vi "subVI_weighted_avg.vi"(9 "input array":dbl[](array[numeric]), 10 "sample":dbl, 11 "no. moving avg.":i32=5) -> (2 "weighted avg.":dbl, 3 "output array":dbl[](array[numeric]))   [LabVIEW 2018]
panel:
  out "array (last n elements first)":dbl[](array[numeric])
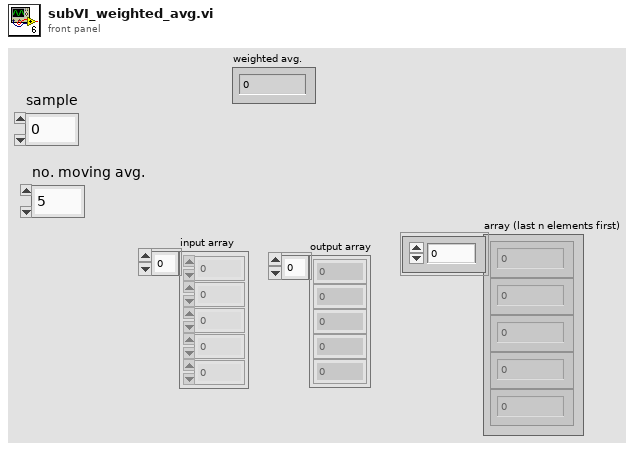
[diagram p1: front panel]
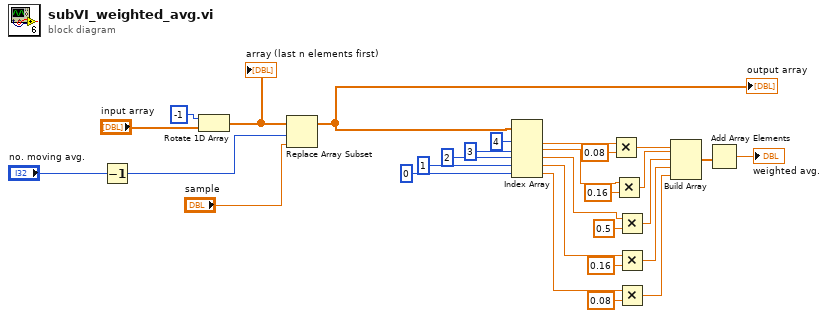
[diagram p0: block diagram]
diagram:
  n1 = Decrement(x="no. moving avg.") -> (x-1=w2:i32)
  n2 = Rotate 1D Array(1:"input array", 2:-1 ("n")) -> (0:w28:dbl[])
  "array (last n elements first)" <- w28
  n3 = Replace Array Subset(array=w28, new element="sample", index=w2) -> (w25:dbl[])
  "output array" <- w25
  n4 = Index Array(array=w25, index #1=4 ("index"), index #2=3 ("index"), index #3=2 ("index"), index #4=1 ("index"), index #5=0 ("index")) -> (element #1=w19:dbl, element #2=w13:dbl, element #3=w12:dbl, element #4=w11:dbl, element #5=w10:dbl)
  n5 = Multiply(x=w19, y=0.08) -> (x*y=w9:dbl)
  n6 = Multiply(x=w13, y=0.16) -> (x*y=w8:dbl)
  n7 = Multiply(x=w12, y=0.5) -> (x*y=w7:dbl)
  n8 = Multiply(x=w11, y=0.16) -> (x*y=w6:dbl)
  n9 = Multiply(x=w10, y=0.08) -> (x*y=w5:dbl)
  n10 = Build Array(w9, w8, w7, w6, w5) -> (w4:dbl[])
  n11 = Add Array Elements(numeric array=w4) -> (sum=→"weighted avg.":dbl)
